vi "IngornePointPanel.vi"() -> ()   [LabVIEW 2019]
uses:
  NozzelUse/Ctrl/Nozzel_Tray_main.ctl
  global/Tray_ArrAndData.vi
  SetPanel/Ctrl/SP_DataCtrl.ctl
  <vilib>/Utility/miscctls.llb/LVPositionTypeDef.ctl
  <vilib>/Utility/miscctls.llb/LVPointTypeDef.ctl
panel:
  out "Numeric":i32
  out "PressALLBtn":string
  in  "Stop Ref":refnum<vi>
  out "NG1":bool[][](array[boolean])
  out "Pass":bool[][](array[boolean])
  out "NG2":bool[][](array[boolean])
  out "Dut":bool[][](array[boolean])
  out "Tray_RefArr":refnum<vi>[](array[refnum])
  out "IngornePointQue":refnum<queue>
  in  "Stop Button":bool
  out "TrayXY":T1
  in  "Tab Control":enum32{"Nozzel3"}(tab)
  out "Enable_Dut 2":bool caption="Enable_Dut"
  out "Enable_NG2 2":bool caption="Enable_Dut"
  in  "Enable_NG1":bool=TRUE caption="Enable_Dut"
  in  "Enable_Pass":bool=TRUE caption="Enable_Dut"
  in  "Enable_NG2":bool=TRUE caption="Enable_Dut"
  in  "Enable_Dut":bool=TRUE
  in  "Btn_Save":bool
  in  "Press_Pass":bool[][](array[boolean])
  in  "Press_Dut":bool[][](array[boolean])
  in  "Press_NG2":bool[][](array[boolean])
  out "Tray Dut Pass":cluster{"Color":u32[][], "Data":string[][]}={"Color"=[[16860, 16860, 16860, 16860, 16860, 16860, 16860, 16860], [16860, 16860, 16860, 16860, 16860, 16860, 16860, 16860], [16860, 16860, 16860, 16860, 16860, 16860, 16860, 16860], [16860, 16860, 16860, 16860, 16860, 16860, 16860, 16860], [16860, 16860, 16860, 16860, 16860, 16860, 16860, 16860], [16860, 16860, 16860, 16860, 16860, 16860, 16860, 16860], [16860, 16860, 16860, 16860, 16860, 16860, 16860, 16860], [16860, 16860, 16860, 16860, 16860, 16860, 16860, 16860], [16860, 16860, 16860, 16860, 16860, 16860, 16860, 16860], [16860, 16860, 16860, 16860, 16860, 16860, 16860, 16860], [16860, 16860, 16860, 16860, 16860, 16860, 16860, 16860], [16860, 16860, 16860, 16860, 16860, 16860, 16860, 16860]], "Data"=[["", "", "", "", "", "", "", ""], ["", "", "", "", "", "", "", ""], ["", "", "", "", "", "", "", ""], ["", "", "", "", "", "", "", ""], ["", "", "", "", "", "", "", ""], ["", "", "", "", "", "", "", ""], ["", "", "", "", "", "", "", ""], ["", "", "", "", "", "", "", ""], ["", "", "", "", "", "", "", ""], ["", "", "", "", "", "", "", ""], ["", "", "", "", "", "", "", ""], ["", "", "", "", "", "", "", ""]]}
  out "Tray Dut":cluster{"Color":u32[][], "Data":string[][]}={"Color"=[[16860, 16860, 16860, 16860, 16860, 16860, 16860, 16860], [16860, 16860, 16860, 16860, 16860, 16860, 16860, 16860], [16860, 16860, 16860, 16860, 16860, 16860, 16860, 16860], [16860, 16860, 16860, 16860, 16860, 16860, 16860, 16860], [16860, 16860, 16860, 16860, 16860, 16860, 16860, 16860], [16860, 16860, 16860, 16860, 16860, 16860, 16860, 16860], [16860, 16860, 16860, 16860, 16860, 16860, 16860, 16860], [16860, 16860, 16860, 16860, 16860, 16860, 16860, 16860], [16860, 16860, 16860, 16860, 16860, 16860, 16860, 16860], [16860, 16860, 16860, 16860, 16860, 16860, 16860, 16860], [16860, 16860, 16860, 16860, 16860, 16860, 16860, 16860], [16860, 16860, 16860, 16860, 16860, 16860, 16860, 16860]], "Data"=[["", "", "", "", "", "", "", ""], ["", "", "", "", "", "", "", ""], ["", "", "", "", "", "", "", ""], ["", "", "", "", "", "", "", ""], ["", "", "", "", "", "", "", ""], ["", "", "", "", "", "", "", ""], ["", "", "", "", "", "", "", ""], ["", "", "", "", "", "", "", ""], ["", "", "", "", "", "", "", ""], ["", "", "", "", "", "", "", ""], ["", "", "", "", "", "", "", ""], ["", "", "", "", "", "", "", ""]]}
  in  "Btn_All_NG1":bool
  in  "Btn_All_Pass":bool
  in  "Btn_All_NG2":bool
  in  "Btn_All_Dut":bool
  in  "NG2 Label":string="NG1(NGA)"
  in  "NG1 Label":string="NG2(NGB)"
  in  "Pass Label":string="PASS"
  in  "Dut Label":string="Dut"
  in  "Tray NG2":cluster{"Color":u32[][], "Data":string[][]}={"Color"=[[16860, 16860, 16860, 16860, 16860, 16860, 16860, 16860], [16860, 16860, 16860, 16860, 16860, 16860, 16860, 16860], [16860, 16860, 16860, 16860, 16860, 16860, 16860, 16860], [16860, 16860, 16860, 16860, 16860, 16860, 16860, 16860], [16860, 16860, 16860, 16860, 16860, 16860, 16860, 16860], [16860, 16860, 16860, 16860, 16860, 16860, 16860, 16860], [16860, 16860, 16860, 16860, 16860, 16860, 16860, 16860], [16860, 16860, 16860, 16860, 16860, 16860, 16860, 16860], [16860, 16860, 16860, 16860, 16860, 16860, 16860, 16860], [16860, 16860, 16860, 16860, 16860, 16860, 16860, 16860], [16860, 16860, 16860, 16860, 16860, 16860, 16860, 16860], [16860, 16860, 16860, 16860, 16860, 16860, 16860, 16860]], "Data"=[["", "", "", "", "", "", "", ""], ["", "", "", "", "", "", "", ""], ["", "", "", "", "", "", "", ""], ["", "", "", "", "", "", "", ""], ["", "", "", "", "", "", "", ""], ["", "", "", "", "", "", "", ""], ["", "", "", "", "", "", "", ""], ["", "", "", "", "", "", "", ""], ["", "", "", "", "", "", "", ""], ["", "", "", "", "", "", "", ""], ["", "", "", "", "", "", "", ""], ["", "", "", "", "", "", "", ""]]}
  in  "Press_NG1":bool[][](array[boolean])
  out "Tray NG":cluster{"Color":u32[][], "Data":string[][]}={"Color"=[[16860, 16860, 16860, 16860, 16860, 16860, 16860, 16860], [16860, 16860, 16860, 16860, 16860, 16860, 16860, 16860], [16860, 16860, 16860, 16860, 16860, 16860, 16860, 16860], [16860, 16860, 16860, 16860, 16860, 16860, 16860, 16860], [16860, 16860, 16860, 16860, 16860, 16860, 16860, 16860], [16860, 16860, 16860, 16860, 16860, 16860, 16860, 16860], [16860, 16860, 16860, 16860, 16860, 16860, 16860, 16860], [16860, 16860, 16860, 16860, 16860, 16860, 16860, 16860], [16860, 16860, 16860, 16860, 16860, 16860, 16860, 16860], [16860, 16860, 16860, 16860, 16860, 16860, 16860, 16860], [16860, 16860, 16860, 16860, 16860, 16860, 16860, 16860], [16860, 16860, 16860, 16860, 16860, 16860, 16860, 16860]], "Data"=[["", "", "", "", "", "", "", ""], ["", "", "", "", "", "", "", ""], ["", "", "", "", "", "", "", ""], ["", "", "", "", "", "", "", ""], ["", "", "", "", "", "", "", ""], ["", "", "", "", "", "", "", ""], ["", "", "", "", "", "", "", ""], ["", "", "", "", "", "", "", ""], ["", "", "", "", "", "", "", ""], ["", "", "", "", "", "", "", ""], ["", "", "", "", "", "", "", ""], ["", "", "", "", "", "", "", ""]]}
  in  "Refresh Set":bool
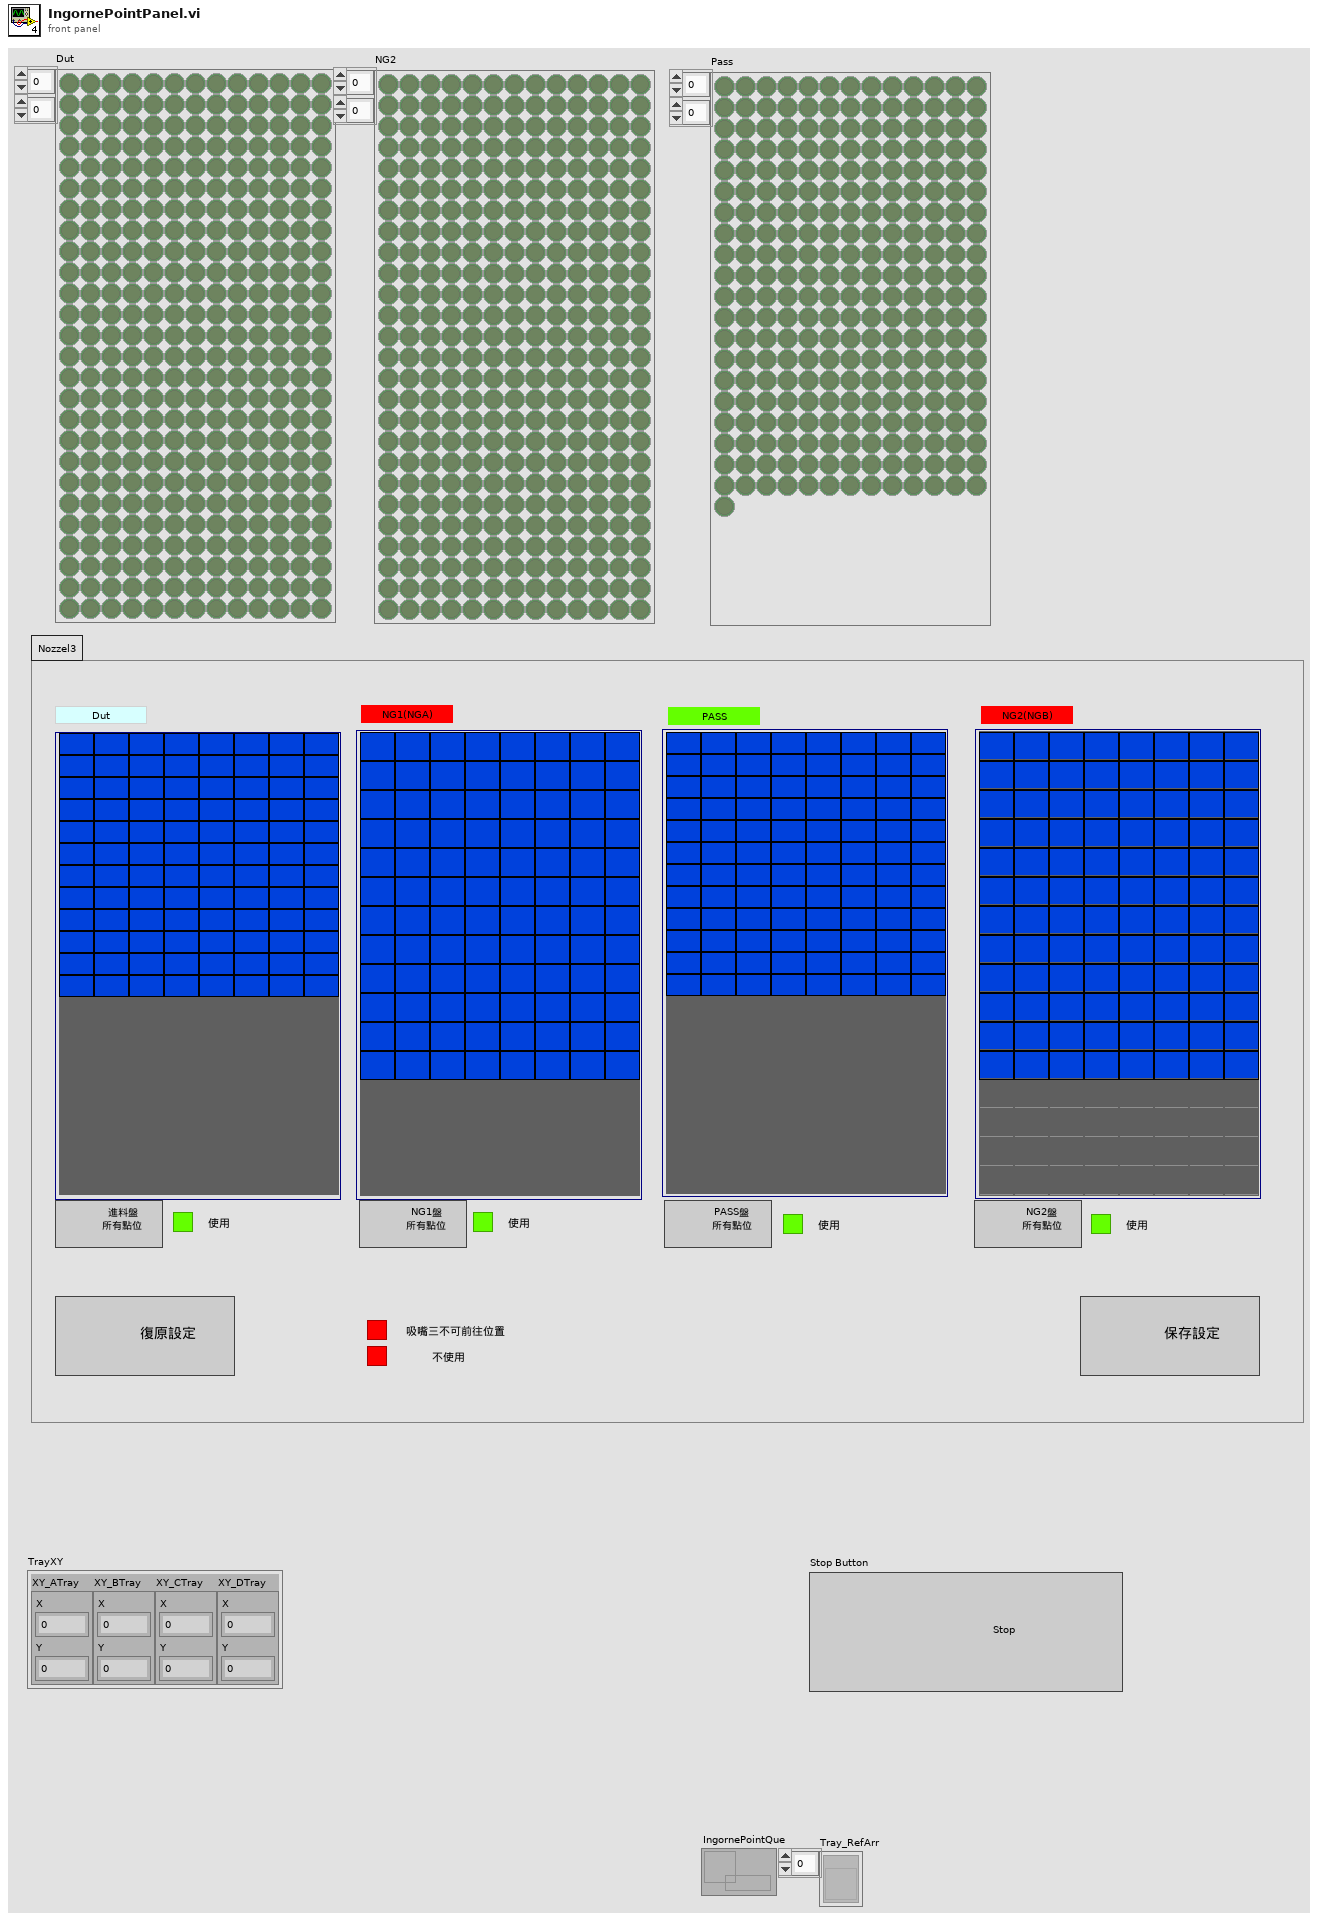
[diagram p1: front panel]
types:
  T1 = cluster{"XY_ATray":cluster{"X":i32, "Y":i32}, "XY_BTray":cluster{"X":i32, "Y":i32}, "XY_CTray":cluster{"X":i32, "Y":i32}, "XY_DTray":cluster{"X":i32, "Y":i32}}
  T2 = typedef "LVPointTypeDef.ctl" = cluster{"Horizontal":i16, "Vertical":i16}
  T3 = typedef "LVPositionTypeDef.ctl" = cluster{"Left":i32, "Top":i32}
  T4 = typedef "Nozzel_Tray_main.ctl" = enum16{"Initial", "Exit", "SetTrayIndex", "SetTRayNumber", "SetTrayAll"}
  T5 = cluster{"BtnArr":refnum<vi>, "BtnRef":refnum<vi>}
  T6 = typedef "SP_DataCtrl.ctl" = enum16{"initial", "save", "load", "write", "read"}
  T7 = cluster{"XY_ATray":cluster{"X":i32, "Y":i32}, "Initial color":u32, "FinalColor":u32}
  T8 = cluster{"XY_DTray":cluster{"X":i32, "Y":i32}, "Initial color":u32, "FinalColor":u32}
  T9 = cluster{"XY_BTray":cluster{"X":i32, "Y":i32}, "Initial color":u32, "FinalColor":u32}
  T10 = cluster{"XY_CTray":cluster{"X":i32, "Y":i32}, "Initial color":u32, "FinalColor":u32}
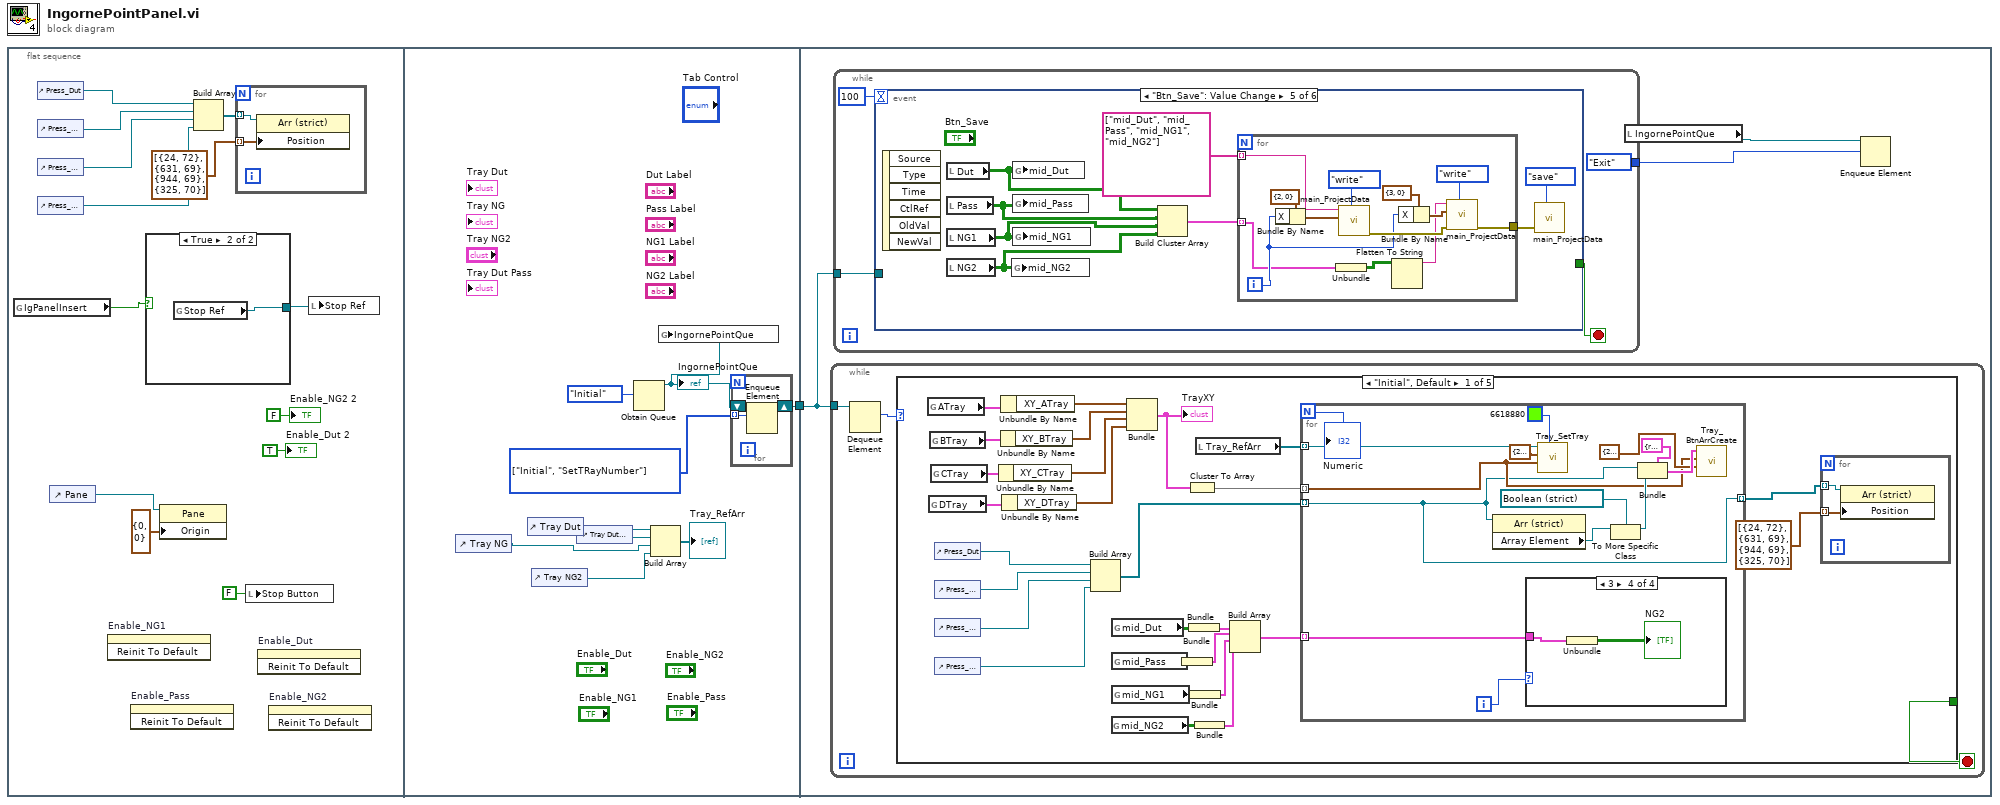
[diagram p0: block diagram]
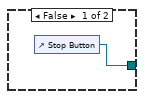
[diagram p2: hidden frame]
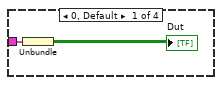
[diagram p3: hidden frame]
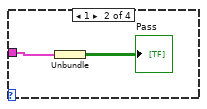
[diagram p4: hidden frame]
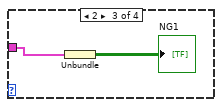
[diagram p5: hidden frame]
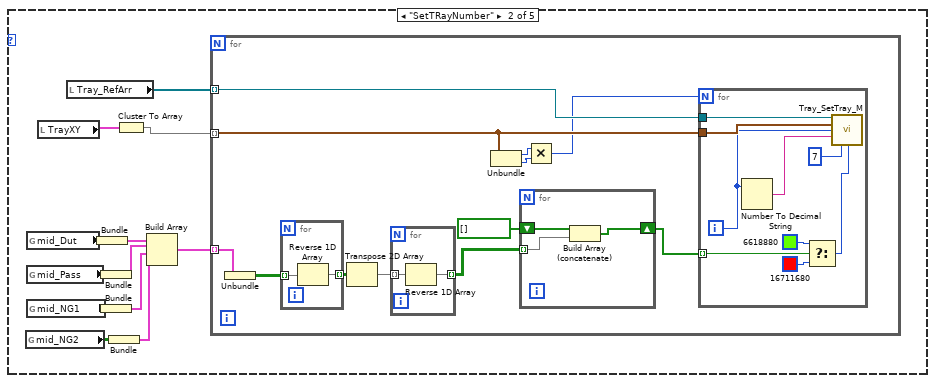
[diagram p6: hidden frame]
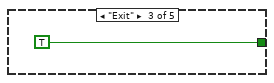
[diagram p7: hidden frame]
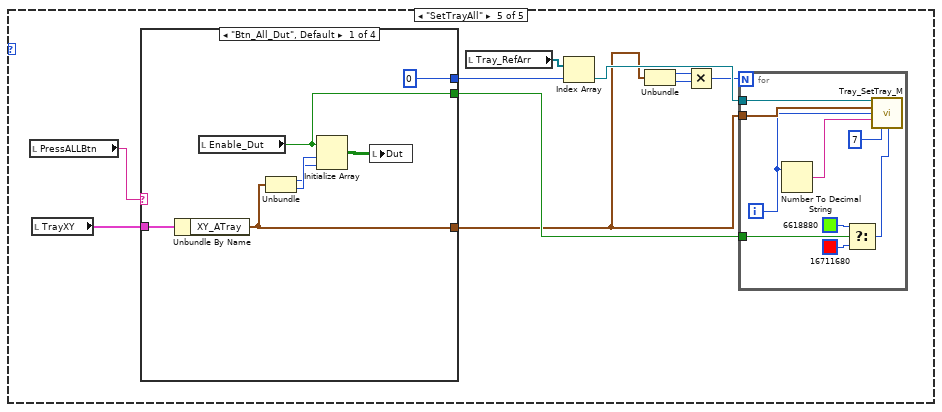
[diagram p9: hidden frame]
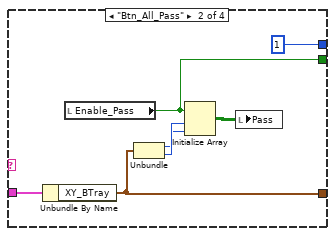
[diagram p10: hidden frame]
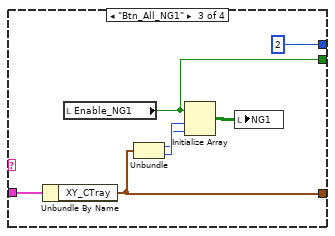
[diagram p11: hidden frame]
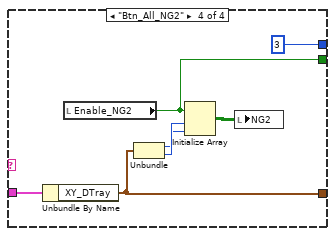
[diagram p12: hidden frame]
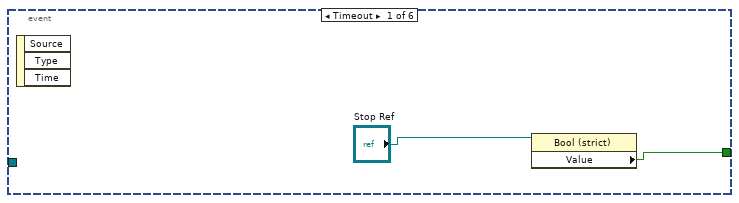
[diagram p13: hidden frame]
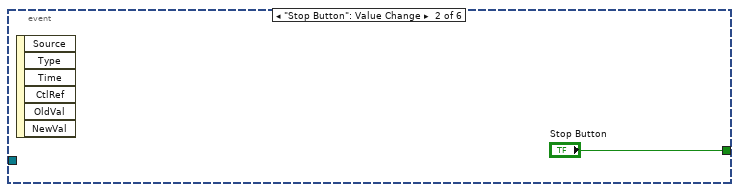
[diagram p14: hidden frame]
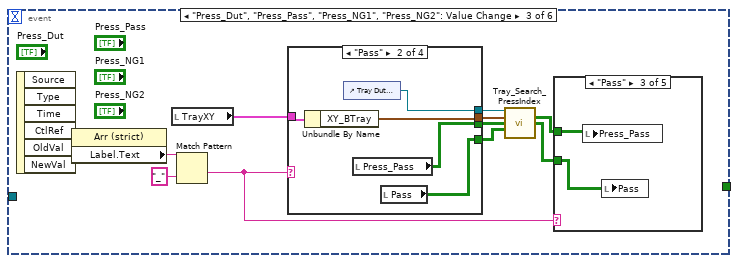
[diagram p15: hidden frame]
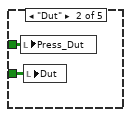
[diagram p17: hidden frame]
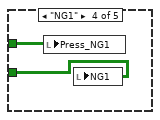
[diagram p18: hidden frame]
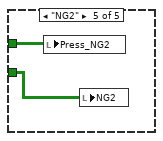
[diagram p19: hidden frame]
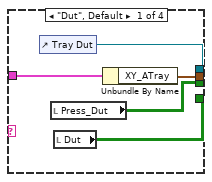
[diagram p20: hidden frame]
diagram:
  n1 = flat-sequence {
    tunnel: [w26] -> w1
    tunnel: w1 -> [w31]
    frame #0 {
      n2 = global read "Tray_ArrAndData.vi" "IgPanelInsert"() -> (w14:bool)
      n3 = control-ref of="Press_Dut"() -> (w6:refnum<vi>)
      n4 = control-ref of="Press_Pass"() -> (w7:refnum<vi>)
      n5 = control-ref of="Press_NG1"() -> (w8:refnum<vi>)
      n6 = control-ref of="Press_NG2"() -> (w9:refnum<vi>)
      n7 = control-ref of="Pane"() -> (w3:refnum<vi>)
      n8 = invoke on="Enable_NG1" class="Bool (strict)" method="Reinit To Default"() -> ()  [unwired: 3 in, 3 out]
      n9 = invoke on="Enable_Pass" class="Bool (strict)" method="Reinit To Default"() -> ()  [unwired: 3 in, 3 out]
      n10 = case shown="True" w14 {
        tunnel: [w17 w18] -> w13
        frame False {
          n11 = control-ref of="Stop Button"() -> (w17:refnum<vi>)
        }
        frame True {
          n12 = global read "Tray_ArrAndData.vi" "Stop Ref"() -> (w18:refnum<vi>)
        }
      }
      n13 = property class="Pane"(reference=w3, "Origin"=T2 {"Horizontal"=0, "Vertical"=0}) -> ()  [unwired: 1 in, 2 out]
      n14 = Build Array(w6, w7, w8, w9) -> (w5:refnum<vi>[])
      n15 = for {
        tunnel: w5 -> [w16] mode=indexing
        tunnel: T3[] [{"Left"=24, "Top"=72}, {"Left"=631, "Top"=69}, {"Left"=944, "Top"=69}, {"Left"=325, "Top"=70}] ("Array") -> [w15] mode=indexing
        n16 = property class="Arr (strict)"(reference=w16, "Position"=w15) -> ()  [unwired: 1 in, 2 out]
      }
      n17 = local write "Stop Button"(FALSE ("Stop Button")) -> ()
      n18 = invoke on="Enable_Dut" class="Bool (strict)" method="Reinit To Default"() -> ()  [unwired: 3 in, 3 out]
      n19 = invoke on="Enable_NG2" class="Bool (strict)" method="Reinit To Default"() -> ()  [unwired: 3 in, 3 out]
      n20 = local write "Stop Ref"(w13) -> ()
      "Enable_NG2 2" <- FALSE ("Enable_NG2 2")
      "Enable_Dut 2" <- TRUE ("Enable_Dut 2")
    }
    frame #1 {
      w20 = T4[] [enum."Initial", enum."SetTRayNumber"] items=["Initial", "Exit", "SetTrayIndex", "SetTRayNumber", "SetTrayAll"]
      n21 = control-ref of="Tray NG"() -> (w24:refnum<vi>)
      n22 = control-ref of="Tray Dut"() -> (w22:refnum<vi>)
      n23 = control-ref of="Tray NG2"() -> (w25:refnum<vi>)
      n24 = control-ref of="Tray Dut Pass"() -> (w23:refnum<vi>)
      n25 = Obtain Queue(element data type=Nozzel_Tray_main."Initial") -> (queue out=w19:refnum<queue>)  [unwired: 4 in, 2 out]
      "IngornePointQue" <- w19
      n26 = Build Array(w22, w23, w24, w25) -> (→"Tray_RefArr":refnum<vi>[])
      n27 = global write "Tray_ArrAndData.vi" "IngornePointQue"(w19) -> ()
      n28 = for {
        shift-right: [w29] -> w26
        shift-left: w19 -> [w30]
        tunnel: w20 -> [w28] mode=indexing
        n29 = Enqueue Element(queue=w30, element=w28) -> (queue out=w29:refnum<queue>)  [unwired: 2 in, 2 out]
      }
    }
    frame #2 {
      n30 = while {
        tunnel: w31 -> [w36]
        stop <- w34 stop-if-true
        n31 = Dequeue Element(queue=w36) -> (element=w35:T4)  [unwired: 2 in, 3 out]
        n32 = case shown="\"Initial\", Default" w35 {
          tunnel: [_ _ TRUE _ _] -> w34
          frame "Initial", Default {
            n33 = global read "Tray_ArrAndData.vi" "ATray"() -> (w60:T7)
            n34 = global read "Tray_ArrAndData.vi" "DTray"() -> (w61:T8)
            n35 = global read "Tray_ArrAndData.vi" "BTray"() -> (w63:T9)
            n36 = global read "Tray_ArrAndData.vi" "CTray"() -> (w62:T10)
            n37 = control-ref of="Press_Dut"() -> (w54:refnum<vi>)
            n38 = control-ref of="Press_Pass"() -> (w53:refnum<vi>)
            n39 = control-ref of="Press_NG1"() -> (w52:refnum<vi>)
            n40 = control-ref of="Press_NG2"() -> (w51:refnum<vi>)
            n41 = Unbundle By Name(w62) -> ("XY_CTray"=w58:cluster{"X":i32, "Y":i32})
            n42 = Unbundle By Name(w63) -> ("XY_BTray"=w59:cluster{"X":i32, "Y":i32})
            n43 = Unbundle By Name(w60) -> ("XY_ATray"=w48:cluster{"X":i32, "Y":i32})
            n44 = Unbundle By Name(w61) -> ("XY_DTray"=w57:cluster{"X":i32, "Y":i32})
            n45 = Build Array(w54, w53, w52, w51) -> (w50:refnum<vi>[])
            n46 = global read "Tray_ArrAndData.vi" "mid_NG2"() -> (w44:bool[][])
            n47 = global read "Tray_ArrAndData.vi" "mid_Dut"() -> (w47:bool[][])
            n48 = global read "Tray_ArrAndData.vi" "mid_Pass"() -> (w46:bool[][])
            n49 = global read "Tray_ArrAndData.vi" "mid_NG1"() -> (w45:bool[][])
            n50 = Bundle("XY_ATray"=w48, "XY_BTray"=w59, "XY_CTray"=w58, "XY_DTray"=w57) -> (w56:T1)  [unwired: 1 in]
            "TrayXY" <- w56
            n51 = Bundle("mid_Pass"=w46) -> (w41:cluster{"mid_Pass":bool[][]})  [unwired: 1 in]
            n52 = Cluster To Array(cluster=w56) -> (array=w55:cluster{"X":i32, "Y":i32}[])
            n53 = Bundle("mid_Dut"=w47) -> (w42:cluster{"mid_Dut":bool[][]})  [unwired: 1 in]
            n54 = Bundle("mid_NG1"=w45) -> (w40:cluster{"mid_NG1":bool[][]})  [unwired: 1 in]
            n55 = Bundle("mid_NG2"=w44) -> (w39:cluster{"mid_NG2":bool[][]})  [unwired: 1 in]
            n56 = local read "Tray_RefArr"() -> (w49:refnum<vi>[])
            n57 = Build Array(w42, w41, w40, w39) -> (w43:cluster{"mid_NG2":bool[][]}[])
            n58 = for {
              N -> [w67]
              tunnel: w49 -> [w78] mode=indexing
              tunnel: w55 -> [w69] mode=indexing
              tunnel: w50 -> [w66] mode=indexing
              tunnel: w43 -> [w68] mode=indexing
              tunnel: [w66] -> w37 mode=indexing
              i -> [w70]
              n59 = property class="Arr (strict)"(reference=w66) -> ("Array Element"=w73:refnum<vi>)  [unwired: 1 in, 2 out]
              n60 = case shown="3" w70 {
                tunnel: w68 -> [w81 w83 w85 w87]
                frame 0, Default {
                  n61 = Unbundle(w81) -> ("mid_NG2"=→"Dut":bool[][])
                }
                frame 1 {
                  n62 = Unbundle(w83) -> ("mid_NG2"=→"Pass":bool[][])
                }
                frame 2 {
                  n63 = Unbundle(w85) -> ("mid_NG2"=→"NG1":bool[][])
                }
                frame 3 {
                  n64 = Unbundle(w87) -> ("mid_NG2"=→"NG2":bool[][])
                }
              }
              n65 = call "Tray_SetTray.vi"("Initial color"=u32 6618880, "GridSize"=w69, "MaxArea"=cluster{"x":u32, "y":u32} {"x"=280, "y"=470}, "Tray in"=w78) -> ()  [unwired: 7 in, 1 out]
              n66 = To More Specific Class(target class=refnum<vi> refnum ("BtnRef"), reference=w73) -> (specific class reference=w72:refnum<vi>)  [unwired: 1 in, 1 out]
              n67 = Bundle(cluster=T5 {"BtnArr"=refnum, "BtnRef"=refnum} ("Refin"), "BtnArr"=w66, "BtnRef"=w72) -> (w75:T5)
              n68 = call "Tray_BtnArrCreate.vi"("MaxArea"=cluster{"x":u32, "y":u32} {"x"=280, "y"=470}, "GridSize"=w69, "Refin"=w75) -> ()  [unwired: 8 in, 1 out]
              "Numeric" <- w67
            }
            n69 = for {
              tunnel: w37 -> [w65] mode=indexing
              tunnel: T3[] [{"Left"=24, "Top"=72}, {"Left"=631, "Top"=69}, {"Left"=944, "Top"=69}, {"Left"=325, "Top"=70}] ("Array") -> [w64] mode=indexing
              n70 = property class="Arr (strict)"(reference=w65, "Position"=w64) -> ()  [unwired: 1 in, 2 out]
            }
          }
          frame "SetTRayNumber" {
            n71 = global read "Tray_ArrAndData.vi" "mid_NG2"() -> (w93:bool[][])
            n72 = global read "Tray_ArrAndData.vi" "mid_Dut"() -> (w96:bool[][])
            n73 = global read "Tray_ArrAndData.vi" "mid_Pass"() -> (w95:bool[][])
            n74 = global read "Tray_ArrAndData.vi" "mid_NG1"() -> (w94:bool[][])
            n75 = local read "TrayXY"() -> (w98:T1)
            n76 = local read "Tray_RefArr"() -> (w99:refnum<vi>[])
            n77 = Bundle("mid_Dut"=w96) -> (w91:cluster{"mid_Dut":bool[][]})  [unwired: 1 in]
            n78 = Bundle("mid_Pass"=w95) -> (w90:cluster{"mid_Pass":bool[][]})  [unwired: 1 in]
            n79 = Bundle("mid_NG1"=w94) -> (w89:cluster{"mid_NG1":bool[][]})  [unwired: 1 in]
            n80 = Bundle("mid_NG2"=w93) -> (w88:cluster{"mid_NG2":bool[][]})  [unwired: 1 in]
            n81 = Cluster To Array(cluster=w98) -> (array=w97:cluster{"X":i32, "Y":i32}[])
            n82 = Build Array(w91, w90, w89, w88) -> (w92:cluster{"mid_NG2":bool[][]}[])
            n83 = for {
              tunnel: w99 -> [w111] mode=indexing
              tunnel: w97 -> [w110] mode=indexing
              tunnel: w92 -> [w101] mode=indexing
              n84 = Unbundle(w101) -> ("mid_NG2"=w100:bool[][])
              n85 = for {
                tunnel: [w115] -> w103 mode=indexing
                tunnel: w100 -> [w114] mode=indexing
                n86 = Reverse 1D Array(array=w114) -> (reversed array=w115:bool[])
              }
              n87 = Transpose 2D Array(2D array=w103) -> (transposed array=w104:bool[][])
              n88 = for {
                tunnel: w104 -> [w113] mode=indexing
                tunnel: [w112] -> w102 mode=indexing
                n89 = Reverse 1D Array(array=w113) -> (reversed array=w112:bool[])
              }
              n90 = Unbundle(w110) -> ("X"=w109:i32, "Y"=w108:i32)
              n91 = for {
                shift-right: [w116] -> w105
                shift-left: bool[] [] -> [w118]
                tunnel: w102 -> [w117] mode=indexing
                n92 = Build Array (concatenate)(w118, w117) -> (w116:bool[])
              }
              n93 = Multiply(x=w109, y=w108) -> (x*y=w107:i32)
              n94 = for {
                N: w107 -> [_]
                tunnel: w110 -> [w126]
                tunnel: w111 -> [w125]
                tunnel: w105 -> [w120] mode=indexing
                i -> [w124]
                n95 = Number To Decimal String(number=w124) -> (decimal integer string=w123:string)  [unwired: 1 in]
                n96 = Select(t=u32 6618880 ("Color Box"), s=w120, f=u32 16711680 ("Color Box")) -> (s? t:f=w119:u32)
                n97 = call "Tray_SetTray_M.vi"("TrayIn"=w125, "GridSize"=w126, "Index Number"=w124, "String"=w123, "Direction"=u16 7, "Color Box"=w119) -> ()  [unwired: 9 in, 1 out]
              }
            }
          }
          frame "Exit" {
          }
          frame "SetTrayIndex" {
          }
          frame "SetTrayAll" {
            n98 = local read "PressALLBtn"() -> (w137:string)
            n99 = local read "TrayXY"() -> (w138:T1)
            n100 = case shown="\"Btn_All_Dut\", Default" w137 {
              tunnel: w138 -> [w154 w161 w168 w175]
              tunnel: [w151 w158 w165 w172] -> w132
              tunnel: [0 1 2 3] -> w135
              tunnel: [w148 w155 w162 w169] -> w133
              frame "Btn_All_Dut", Default {
                n101 = Unbundle By Name(w154) -> ("XY_ATray"=w151:cluster{"X":i32, "Y":i32})
                n102 = local read "Enable_Dut"() -> (w148:bool)
                n103 = Unbundle(w151) -> ("X"=w149:i32, "Y"=w150:i32)
                n104 = Initialize Array(w148, w150, w149) -> (w152:bool[][])
                n105 = local write "Dut"(w152) -> ()
              }
              frame "Btn_All_Pass" {
                n106 = Unbundle By Name(w161) -> ("XY_BTray"=w158:cluster{"X":i32, "Y":i32})
                n107 = local read "Enable_Pass"() -> (w155:bool)
                n108 = Unbundle(w158) -> ("X"=w156:i32, "Y"=w157:i32)
                n109 = Initialize Array(w155, w157, w156) -> (w159:bool[][])
                n110 = local write "Pass"(w159) -> ()
              }
              frame "Btn_All_NG1" {
                n111 = Unbundle By Name(w168) -> ("XY_CTray"=w165:cluster{"X":i32, "Y":i32})
                n112 = local read "Enable_NG1"() -> (w162:bool)
                n113 = Unbundle(w165) -> ("X"=w163:i32, "Y"=w164:i32)
                n114 = Initialize Array(w162, w164, w163) -> (w166:bool[][])
                n115 = local write "NG1"(w166) -> ()
              }
              frame "Btn_All_NG2" {
                n116 = Unbundle By Name(w175) -> ("XY_DTray"=w172:cluster{"X":i32, "Y":i32})
                n117 = local read "Enable_NG2"() -> (w169:bool)
                n118 = Unbundle(w172) -> ("X"=w170:i32, "Y"=w171:i32)
                n119 = Initialize Array(w169, w171, w170) -> (w173:bool[][])
                n120 = local write "NG2"(w173) -> ()
              }
            }
            n121 = local read "Tray_RefArr"() -> (w136:refnum<vi>[])
            n122 = Index Array(array=w136, index=w135) -> (element=w134:refnum<vi>)
            n123 = Unbundle(w132) -> ("X"=w131:i32, "Y"=w130:i32)
            n124 = Multiply(x=w131, y=w130) -> (x*y=w129:i32)
            n125 = for {
              N: w129 -> [_]
              tunnel: w132 -> [w146]
              tunnel: w134 -> [w145]
              tunnel: w133 -> [w140]
              i -> [w144]
              n126 = Number To Decimal String(number=w144) -> (decimal integer string=w143:string)  [unwired: 1 in]
              n127 = Select(t=u32 6618880 ("Color Box"), s=w140, f=u32 16711680 ("Color Box")) -> (s? t:f=w139:u32)
              n128 = call "Tray_SetTray_M.vi"("TrayIn"=w145, "GridSize"=w146, "Index Number"=w144, "String"=w143, "Direction"=u16 7, "Color Box"=w139) -> ()  [unwired: 9 in, 1 out]
            }
          }
        }
      }
      n129 = while {
        tunnel: [Nozzel_Tray_main."Exit" ("element")] -> w32
        tunnel: w31 -> [w177]
        stop <- w179 stop-if-true
        n130 = event shown="[4] \"Btn_Save\": Value Change" {
          selector: _ -> [_ _ _ _ _ _]
          dyn-events: _ -> [_ _ _ _ _ _]
          timeout: 100 -> [_ _ _ _ _ _]
          tunnel: [w180 "Stop Button" _ _ _ _] -> w179
          tunnel: w177 -> [_ _ _ w223 _ w249]
          event Timeout {
            n131 = event-data() -> ()  [unwired: 1 in, 3 out]
            n132 = property class="Bool (strict)"(reference="Stop Ref") -> ("Value"=w180:bool)  [unwired: 1 in, 2 out]
          }
          event "Stop Button": Value Change {
            n133 = event-data() -> ()  [unwired: 1 in, 6 out]
          }
          event "Press_Dut", "Press_Pass", "Press_NG1", "Press_NG2": Value Change {
            n134 = event-data() -> ("CtlRef"=w186:refnum<vi>)  [unwired: 1 in, 5 out]
            n135 = property class="Arr (strict)"(reference=w186) -> ("Label.Text"=w185:string)  [unwired: 1 in, 2 out]
            n136 = local read "TrayXY"() -> (w187:T1)
            n137 = Match Pattern(string=w185, regular expression="_") -> (after substring=w183:string)  [unwired: 1 in, 3 out]
            n138 = case shown="\"Pass\"" w183 {
              tunnel: [w206 w211 w216 w221] -> w193
              tunnel: [w205 w208 w212 w218] -> w190
              tunnel: [w204 w207 w213 w217] -> w189
              tunnel: [w203 w209 w214 w219] -> w188
              tunnel: w187 -> [w202 w210 w215 w220]
              frame "Dut", Default {
                n139 = control-ref of="Tray Dut"() -> (w206:refnum<vi>)
                n140 = local read "Press_Dut"() -> (w205:bool[][])
                n141 = local read "Dut"() -> (w204:bool[][])
                n142 = Unbundle By Name(w202) -> ("XY_ATray"=w203:cluster{"X":i32, "Y":i32})
              }
              frame "Pass" {
                n143 = Unbundle By Name(w210) -> ("XY_BTray"=w209:cluster{"X":i32, "Y":i32})
                n144 = control-ref of="Tray Dut Pass"() -> (w211:refnum<vi>)
                n145 = local read "Press_Pass"() -> (w208:bool[][])
                n146 = local read "Pass"() -> (w207:bool[][])
              }
              frame "NG1" {
                n147 = local read "Press_NG1"() -> (w212:bool[][])
                n148 = Unbundle By Name(w215) -> ("XY_CTray"=w214:cluster{"X":i32, "Y":i32})
                n149 = control-ref of="Tray NG"() -> (w216:refnum<vi>)
                n150 = local read "NG1"() -> (w213:bool[][])
              }
              frame "NG2" {
                n151 = local read "Press_NG2"() -> (w218:bool[][])
                n152 = Unbundle By Name(w220) -> ("XY_DTray"=w219:cluster{"X":i32, "Y":i32})
                n153 = control-ref of="Tray NG2"() -> (w221:refnum<vi>)
                n154 = local read "NG2"() -> (w217:bool[][])
              }
            }
            n155 = call "Tray_Search_PressIndex.vi"("TrayIn"=w193, "XY_DTray"=w188, "Press_Arr"=w190, "Record_Arr In"=w189) -> ("Press_Arr Out"=w192:bool[][], "Record_Arr Out"=w191:bool[][])  [unwired: 10 in]
            n156 = case shown="\"Pass\"" w183 {
              tunnel: w192 -> [_ w195 w196 w199 w201]
              tunnel: w191 -> [_ w194 w197 w198 w200]
              frame "False", Default {
              }
              frame "Dut" {
                n157 = local write "Press_Dut"(w195) -> ()
                n158 = local write "Dut"(w194) -> ()
              }
              frame "Pass" {
                n159 = local write "Press_Pass"(w196) -> ()
                n160 = local write "Pass"(w197) -> ()
              }
              frame "NG1" {
                n161 = local write "Press_NG1"(w199) -> ()
                n162 = local write "NG1"(w198) -> ()
              }
              frame "NG2" {
                n163 = local write "Press_NG2"(w201) -> ()
                n164 = local write "NG2"(w200) -> ()
              }
            }
          }
          event "Refresh Set": Value Change {
            w222 = T4[] [enum."Initial", enum."SetTRayNumber"] items=["Initial", "Exit", "SetTrayIndex", "SetTRayNumber", "SetTrayAll"]
            n165 = event-data() -> ()  [unwired: 1 in, 6 out]
            n166 = for {
              shift-right: [w225] -> _
              shift-left: w223 -> [w226]
              tunnel: w222 -> [w224] mode=indexing
              n167 = Enqueue Element(queue=w226, element=w224) -> (queue out=w225:refnum<queue>)  [unwired: 2 in, 2 out]
            }
          }
          event "Btn_Save": Value Change {
            n168 = event-data() -> ()  [unwired: 1 in, 6 out]
            n169 = local read "Dut"() -> (w234:bool[][])
            n170 = local read "Pass"() -> (w233:bool[][])
            n171 = local read "NG1"() -> (w232:bool[][])
            n172 = local read "NG2"() -> (w231:bool[][])
            n173 = global write "Tray_ArrAndData.vi" "mid_NG2"(w231) -> ()
            n174 = global write "Tray_ArrAndData.vi" "mid_Dut"(w234) -> ()
            n175 = global write "Tray_ArrAndData.vi" "mid_Pass"(w233) -> ()
            n176 = global write "Tray_ArrAndData.vi" "mid_NG1"(w232) -> ()
            n177 = Build Cluster Array(w234, w233, w232, w231) -> (w230:cluster{"NG2":bool[][]}[])
            n178 = for {
              tunnel: w230 -> [w238] mode=indexing
              tunnel: string[] ["mid_Dut", "mid_Pass", "mid_NG1", "mid_NG2"] -> [w244] mode=indexing
              tunnel: [w235] -> w227
              i -> [w239]
              n179 = Bundle By Name(cluster=cluster{"Y":i32, "X":i32} {"Y"=2, "X"=0} ("Index"), "X"=w239) -> (w245:cluster{"Y":i32, "X":i32})
              n180 = Unbundle(w238) -> ("NG2"=w237:bool[][])
              n181 = call "main_ProjectData.vi"("Enum"=SP_DataCtrl."write", "Index"=w245, "DataIn"=w244) -> ("error out"=w240:errorcluster)  [unwired: 6 in, 2 out]
              n182 = Flatten To String(anything=w237) -> (data string=w236:string)  [unwired: 3 in, 2 out]
              n183 = Bundle By Name(cluster=cluster{"Y":i32, "X":i32} {"Y"=3, "X"=0} ("Index"), "X"=w239) -> (w241:cluster{"Y":i32, "X":i32})
              n184 = call "main_ProjectData.vi"("Enum"=SP_DataCtrl."write", "error in"=w240, "Index"=w241, "DataIn"=w236) -> ("error out"=w235:errorcluster)  [unwired: 5 in, 2 out]
            }
            n185 = call "main_ProjectData.vi"("Enum"=SP_DataCtrl."save", "error in"=w227) -> ()  [unwired: 7 in, 3 out]
          }
          event "Btn_All_Dut", "Btn_All_NG2", "Btn_All_Pass", "Btn_All_NG1": Value Change {
            n186 = event-data() -> ("CtlRef"=w250:refnum<vi>)  [unwired: 1 in, 5 out]
            n187 = flat-sequence {
              tunnel: w250 -> [w253]
              tunnel: [Nozzel_Tray_main."SetTrayAll" ("element")] -> w248
              frame #0 {
                n188 = property class="Bool"(reference=w253) -> ("Label.Text"=→"PressALLBtn":string)  [unwired: 1 in, 2 out]
              }
            }
            n189 = Enqueue Element(queue=w249, element=w248) -> ()  [unwired: 2 in, 3 out]
          }
        }
      }
      n190 = local read "IngornePointQue"() -> (w33:refnum<queue>)
      n191 = Enqueue Element(queue=w33, element=w32) -> ()  [unwired: 2 in, 3 out]
    }
  }
